vi "detect pattern.vi"(10 "pattern matching phrase":string, 11 "input bitstream":i8[](array[numeric])) -> (3 "string":string)   [LabVIEW 2013]
panel:
  in  "QAM system parameters":T1
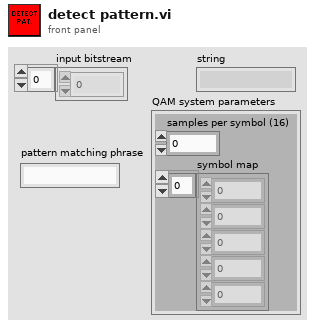
[diagram p1: front panel]
types:
  T1 = cluster{"samples per symbol (16)":i32, "symbol map":cdb[]}
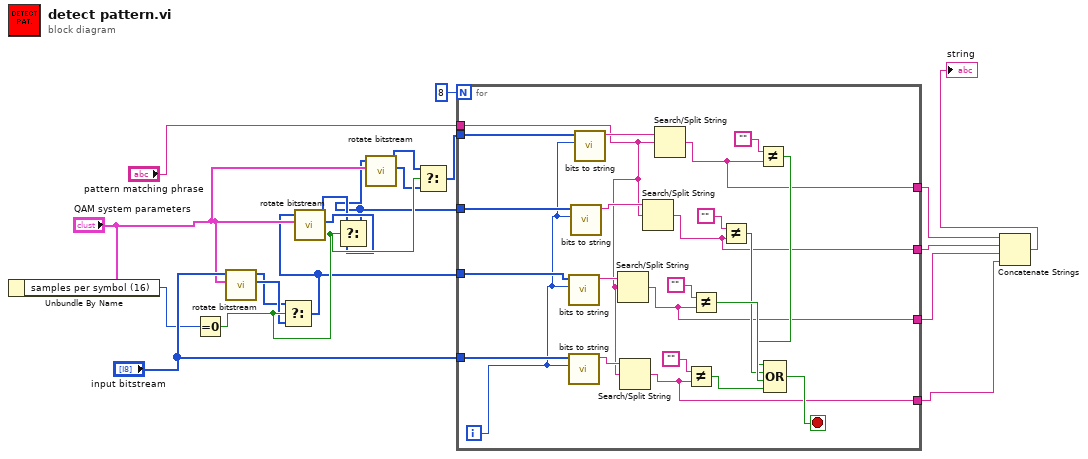
[diagram p0: block diagram]
diagram:
  n1 = Unbundle By Name("QAM system parameters") -> ("samples per symbol (16)"=w11:i32)
  n2 = Equal To 0?(x=w11) -> (x = 0?=w10:bool)
  n3 = call "rotate bitstream.vi"("QAM system parameters"="QAM system parameters", "input bit stream"="input bitstream") -> ("output bit stream rotated using QAM parameters"=w9:i8[], "output bit stream rotated M-ary 4"=w8:i8[])  [unwired: 8 in]
  n4 = Select(t=w8, s=w10, f=w9) -> (s? t:f=w7:i8[])
  n5 = call "rotate bitstream.vi"("QAM system parameters"="QAM system parameters", "input bit stream"=w7) -> ("output bit stream rotated using QAM parameters"=w6:i8[], "output bit stream rotated M-ary 4"=w5:i8[])  [unwired: 8 in]
  n6 = Select(t=w5, s=w10, f=w6) -> (s? t:f=w4:i8[])
  n7 = call "rotate bitstream.vi"("QAM system parameters"="QAM system parameters", "input bit stream"=w4) -> ("output bit stream rotated using QAM parameters"=w2:i8[], "output bit stream rotated M-ary 4"=w3:i8[])  [unwired: 8 in]
  n8 = Select(t=w3, s=w10, f=w2) -> (s? t:f=w1:i8[])
  n9 = for {
    N: 8 -> [_]
    tunnel: w1 -> [w43]
    tunnel: w4 -> [w42]
    tunnel: w7 -> [w41]
    tunnel: "input bitstream" -> [w40]
    tunnel: "pattern matching phrase" -> [w26]
    tunnel: [w24] -> w17
    tunnel: [w23] -> w16
    tunnel: [w22] -> w15
    tunnel: [w21] -> w14
    i -> [w25]
    stop <- w31 stop-if-true
    n10 = call "bits to string.vi"("shift index"=w25, "bit stream"=w41) -> ("string"=w28:string)  [unwired: 9 in]
    n11 = call "bits to string.vi"("shift index"=w25, "bit stream"=w40) -> ("string"=w29:string)  [unwired: 9 in]
    n12 = call "bits to string.vi"("shift index"=w25, "bit stream"=w42) -> ("string"=w27:string)  [unwired: 9 in]
    n13 = call "bits to string.vi"("shift index"=w25, "bit stream"=w43) -> ("string"=w30:string)  [unwired: 9 in]
    n14 = Search/Split String(string=w28, search string/char (-)=w26) -> (match + rest of string=w22:string)  [unwired: 1 in, 2 out]
    n15 = Search/Split String(string=w29, search string/char (-)=w26) -> (match + rest of string=w21:string)  [unwired: 1 in, 2 out]
    n16 = Search/Split String(string=w27, search string/char (-)=w26) -> (match + rest of string=w23:string)  [unwired: 1 in, 2 out]
    n17 = Search/Split String(string=w30, search string/char (-)=w26) -> (match + rest of string=w24:string)  [unwired: 1 in, 2 out]
    n18 = Not Equal?(x="", y=w21) -> (x != y?=w35:bool)
    n19 = Not Equal?(x="", y=w22) -> (x != y?=w34:bool)
    n20 = Not Equal?(x="", y=w23) -> (x != y?=w33:bool)
    n21 = Not Equal?(x="", y=w24) -> (x != y?=w32:bool)
    n22 = Compound Arithmetic op=OR(w32, w33, w34, w35) -> (w31:bool)
  }
  n23 = Concatenate Strings(w17, w16, w15, w14) -> (→"string":string)
